vi "Version.vi"(8 "error in (no error)":errorcluster, 11 "CLI Client in":refnum<class "JFrog CLI.lvclass">) -> (0 "error out":errorcluster, 1 "Ellapsed Time [Sec]":dbl, 2 "Version":string, 3 "CLI Client out":refnum<class "JFrog CLI.lvclass">)   [LabVIEW 2015, in "JFrog CLI.lvclass"]
uses:
  JFrog CLI.lvclass
  JFrog CLI.lvclass/JFrog CLI.ctl
panel:
  out "command line":string
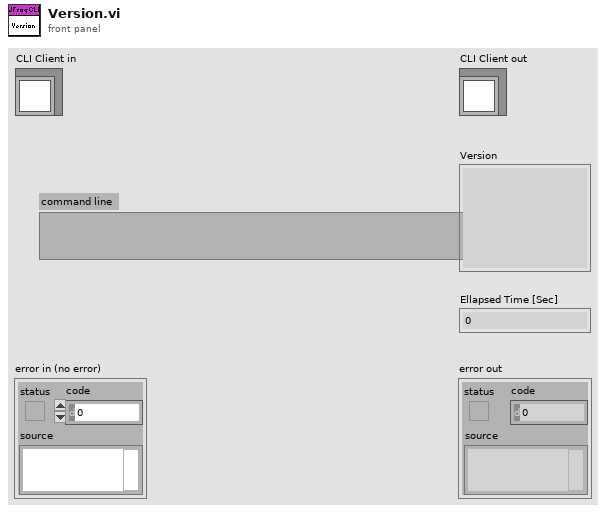
[diagram p1: front panel]
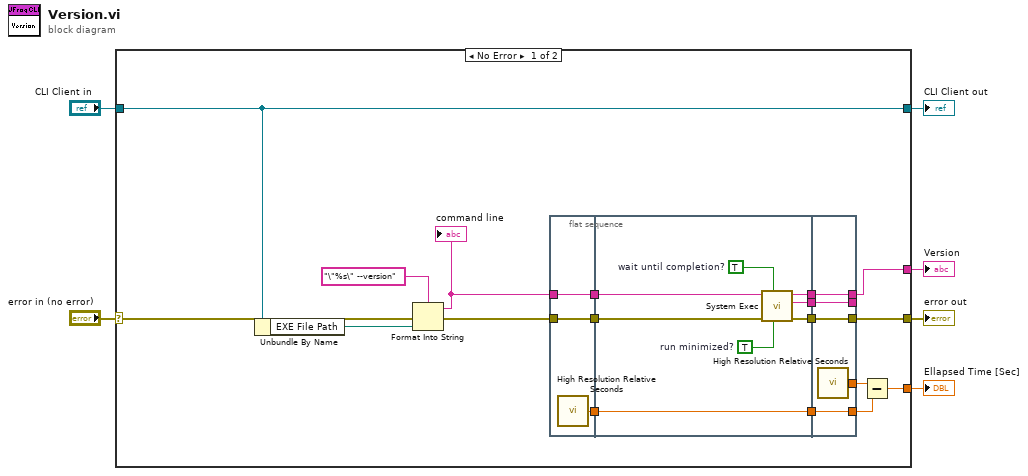
[diagram p0: block diagram]
diagram:
  n1 = case shown="No Error" "error in (no error)" {
    selector: "error in (no error)" -> [w10 w42]
    tunnel: [w9 w42] -> w5
    tunnel: [w11 w41] -> w3
    tunnel: "CLI Client in" -> [w11 w41]
    tunnel: [w8 _] -> w2
    tunnel: [w7 _] -> w1
    frame No Error {
      n2 = Unbundle By Name(w11) -> ("EXE File Path"=w14:path)
      n3 = Format Into String(format string="\"%s\" --version", error in=w10, w14) -> (resulting string=w15:string, error out=w17:errorcluster)  [unwired: 1 in]
      "command line" <- w15
      n4 = flat-sequence {
        tunnel: w15 -> [w26]
        tunnel: w17 -> [w27]
        tunnel: [w27] -> w24
        tunnel: [w26] -> w23
        tunnel: [w25] -> w22
        tunnel: [w35] -> w21
        tunnel: [w31] -> w20
        tunnel: [w30] -> w19
        tunnel: w24 -> [w34]
        tunnel: w23 -> [w29]
        tunnel: [w28] -> w18
        tunnel: w22 -> [w28]
        tunnel: [w38] -> _
        tunnel: [w39] -> w7
        tunnel: [w40] -> w9
        tunnel: w21 -> [w40]
        tunnel: w20 -> [w39]
        tunnel: w19 -> [w38]
        tunnel: [w37] -> w13
        tunnel: [w36] -> w12
        tunnel: w18 -> [w36]
        frame #0 {
          n5 = call <vilib>:"High Resolution Relative Seconds.vi"() -> ("relative seconds"=w25:dbl)
        }
        frame #1 {
          w32 = TRUE  # run minimized?
          w33 = TRUE  # wait until completion?
          n6 = call <vilib>:"System Exec.vi"("run minimized? (F)"=w32, "wait until completion? (T)"=w33, "error in (no error)"=w34, "command line"=w29) -> ("error out"=w35:errorcluster, "standard error"=w30:string, "standard output"=w31:string)  [unwired: 4 in, 1 out]
        }
        frame #2 {
          n7 = call <vilib>:"High Resolution Relative Seconds.vi"() -> ("relative seconds"=w37:dbl)
        }
      }
      n8 = Subtract(x=w13, y=w12) -> (x-y=w8:dbl)
    }
    frame Error {
    }
  }
  "error out" <- w5
  "CLI Client out" <- w3
  "Ellapsed Time [Sec]" <- w2
  "Version" <- w1
